vi "UPdate MaskROIDataEntry.vi"(0 "AllProcessSettingIn":T1[](array[typedef]), 11 "error in (no error)":errorcluster) -> (4 "AllProcessSettingOut":T1[](array[typedef]), 6 "ROIName":string[](array[string]), 8 "Enabled/Disabled":bool, 10 "Color Box":u32, 15 "error out":errorcluster)   [LabVIEW 2019]
uses:
  Controls/Process_Type.ctl
  Controls/MaskROIList_Action.ctl
  Controls/MaskParam_Type.ctl
  Controls/Process_Setting.ctl
  Ctrl/VisionProcessName.ctl
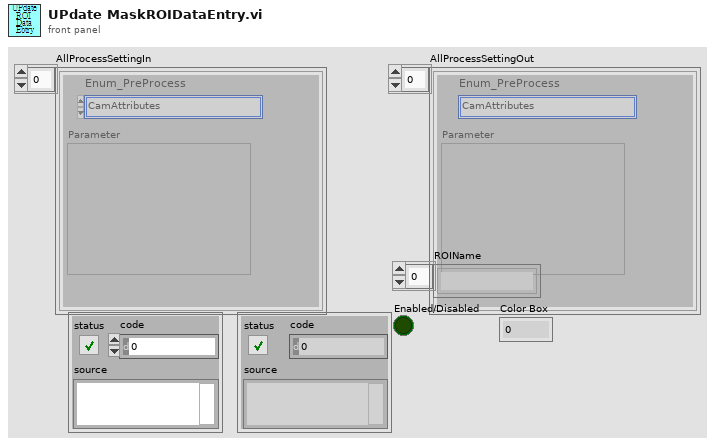
[diagram p1: front panel]
types:
  T1 = typedef "Process_Setting.ctl" = cluster{"Enum_PreProcess":T2, "Parameter":string}
  T2 = typedef "VisionProcessName.ctl" = enum16{"*CamParameter*", "CamAttributes", "*Preprocess*", "CG_Brightness", "C_Plane Extraction", "C_Threshold", "G_Lookup Table", "G_Threshold"}
  T3 = typedef "Process_Type.ctl" = enum16{"None", "ExtractPlane", "BinaryMono", "Operators", "GrayMorphology", "Filters", "Lookup Table", "Particle Filter", "Mask"}
  T4 = typedef "MaskROIList_Action.ctl" = enum16{"initialize", "SaveAll", "ReadAll", "Append", "Replace", "DeleteIndex"}
  T5 = typedef "MaskParam_Type.ctl" = cluster{"Function":enum16{"Inside", "Outside"}, "ROI List":i32, "ROI":cluster{"Global Rectangle":i32[], "Contours":cluster{"Contour Type":u32, "ROI Type":u32, "Points":i32[]}[]}[], "Creat ROI":bool, "Delete ROI":bool, "Enabled/Disabled":bool, "Color Box":u32, "Last Mouse Position":cluster{"X":i32, "Y":i32}}
  T6 = cluster{"Global Rectangle":i32[], "Contours":cluster{"Contour Type":u32, "ROI Type":u32, "Points":i32[]}[]}[]
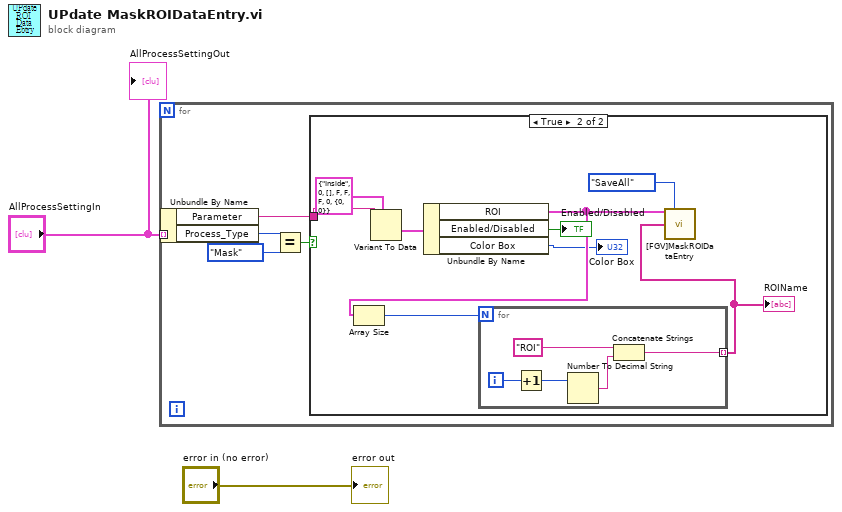
[diagram p0: block diagram]
diagram:
  n1 = for {
    tunnel: "AllProcessSettingIn" -> [w7] mode=indexing
    n2 = Unbundle By Name(w7) -> ("Parameter"=w3:string, "Process_Type"=w6:T3)
    n3 = Equal?(x=w6, y=Process_Type."Mask") -> (x = y?=w4:bool)
    n4 = case shown="True" w4 {
      tunnel: w3 -> [_ w16]
      frame False {
      }
      frame True {
        n5 = Variant To Data(type=T5 {"Function"=enum."Inside", "ROI List"=0, "ROI"=[], "Creat ROI"=FALSE, "Delete ROI"=FALSE, "Enabled/Disabled"=FALSE, "Color Box"=0, "Last Mouse Position"={"X"=0, "Y"=0}} ("MaskParam"), Variant=w16) -> (data=w14:T5)  [unwired: 1 in, 1 out]
        n6 = Unbundle By Name(w14) -> ("ROI"=w12:T6, "Enabled/Disabled"=→"Enabled/Disabled":bool, "Color Box"=→"Color Box":u32)
        n7 = Array Size(array=w12) -> (size(s)=w11:i32)
        n8 = for {
          N: w11 -> [_]
          tunnel: [w17] -> w10 mode=indexing
          i -> [w21]
          n9 = Increment(x=w21) -> (x+1=w20:i32)
          n10 = Number To Decimal String(number=w20) -> (decimal integer string=w19:string)  [unwired: 1 in]
          n11 = Concatenate Strings("ROI", w19) -> (w17:string)
        }
        "ROIName" <- w10
        n12 = call "[FGV]MaskROIDataEntry.vi"("ROI"=w12, "[FGV]MaskROIList_Action"=MaskROIList_Action."SaveAll", "ROINameIn"=w10) -> ()  [unwired: 10 in, 3 out]
      }
    }
  }
  "error out" <- "error in (no error)"
  "AllProcessSettingOut" <- "AllProcessSettingIn"
